vi "4155C PulsedStressV Config SMUs.vi"(0 "VISA resource name in":refnum<visa-resource-name>, 1 "Gate ON voltage":dbl min=-100.0 max=100.0 step=0.005 format="%.3f", 3 "Gate Standby":bool, 5 "Pulse period 2":dbl=0.05 min=0.005 max=1.0 step=0.0001 format="%.4f", 6 "SMU4":cluster{"on/off":bool, "Voltage":dbl} {"Voltage" min=-100.0 max=100.0 format="%.2f"}, 7 "Pulse width 2":dbl=0.0005 min=0.0005 max=0.1 step=0.0001 format="%.4f", 8 "Base voltage 2":dbl format="%^.4e", 11 "error in (no error)":errorcluster, 12 "Drain Voltage":dbl min=-100.0 max=100.0 step=0.005 format="%.3f", 14 "Drain Standby":bool) -> (4 "VISA Resource Name out":refnum<visa-resource-name>, 15 "error out":errorcluster)   [LabVIEW 2016]
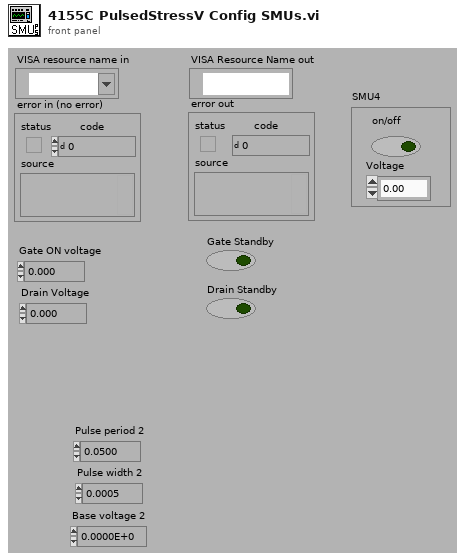
[diagram p1: front panel]
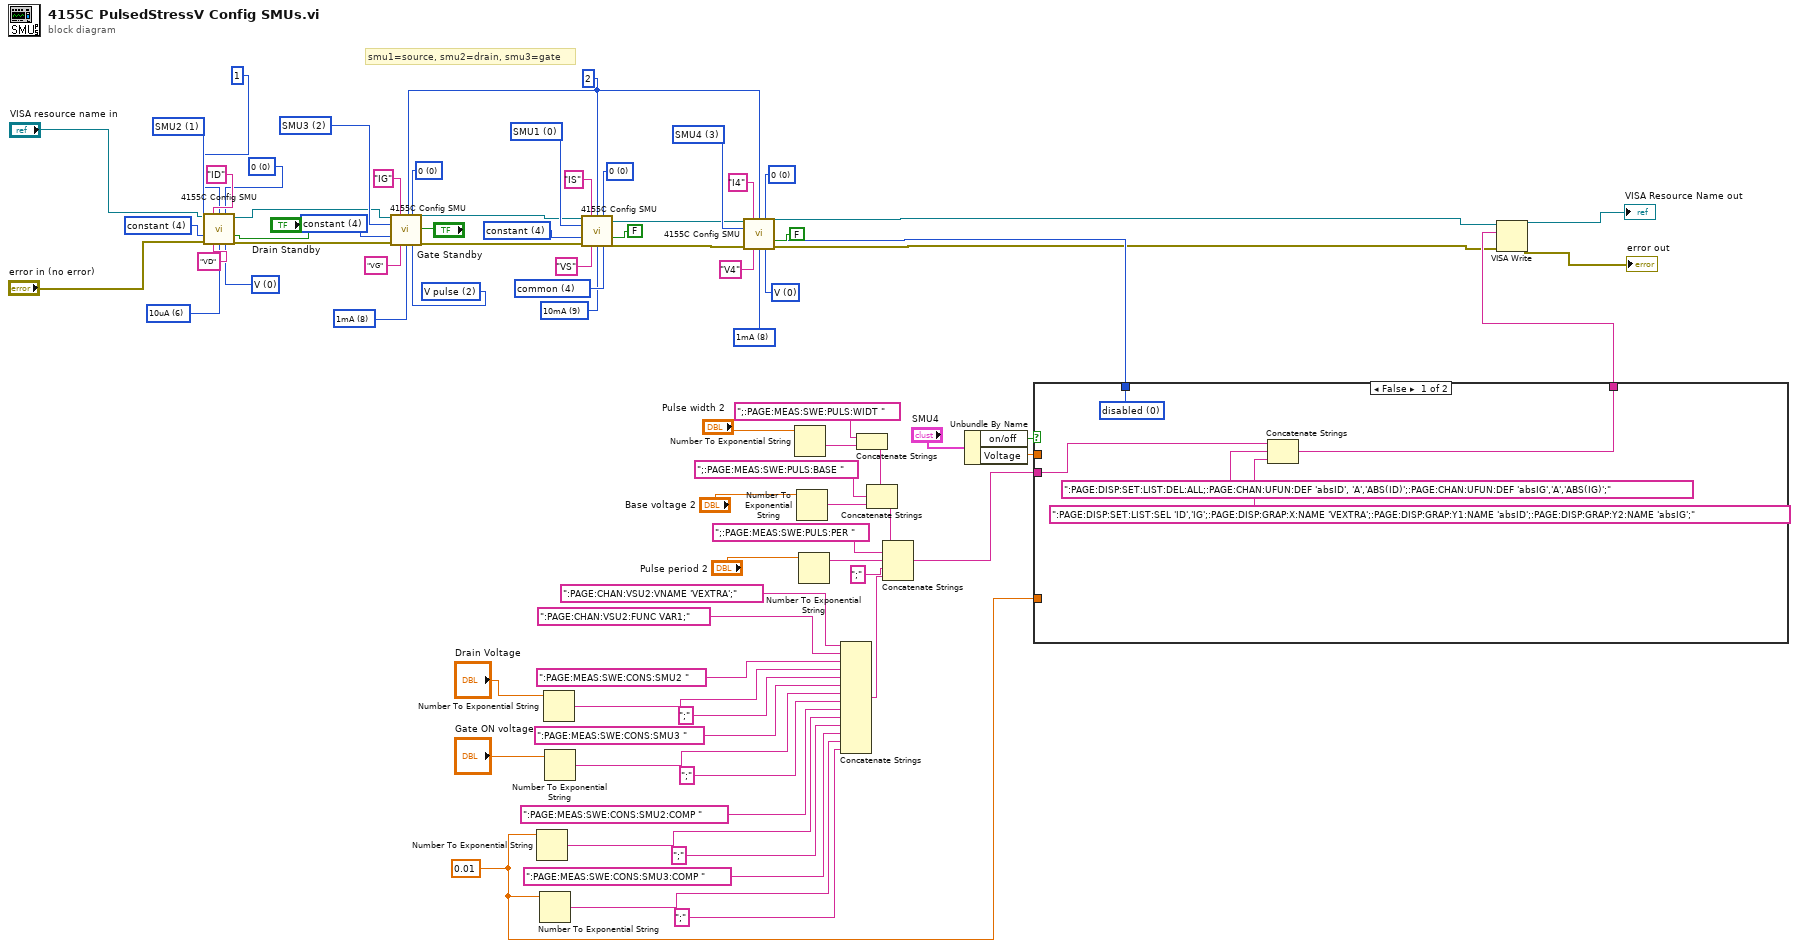
[diagram p0: block diagram]
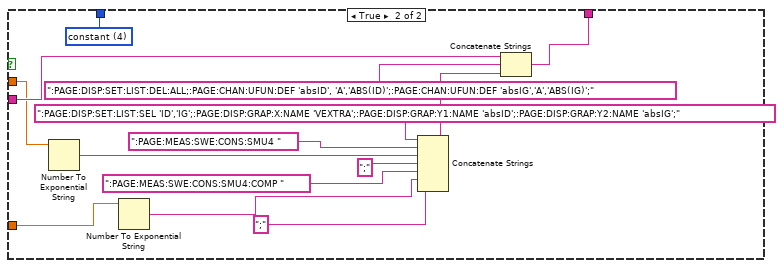
[diagram p2: hidden frame]
diagram:
  w13 = u8 6 items=["10pA  ", "100pA  ", "1nA  ", "10nA", "100nA", "1uA", "10uA", "100uA", "1mA", "10mA", "100mA", "1A"] ("Range")
  w18 = u8 8 items=["10pA  ", "100pA  ", "1nA  ", "10nA", "100nA", "1uA", "10uA", "100uA", "1mA", "10mA", "100mA", "1A"] ("Range")
  w22 = u8 8 items=["10pA  ", "100pA  ", "1nA  ", "10nA", "100nA", "1uA", "10uA", "100uA", "1mA", "10mA", "100mA", "1A"] ("Range")
  w23 = u32 2 items=["V  ", "I  ", "V pulse  ", "I pulse  ", "  common  "] ("mode")
  w21 = 2
  w24 = u8 9 items=["10pA  ", "100pA  ", "1nA  ", "10nA", "100nA", "1uA", "10uA", "100uA", "1mA", "10mA", "100mA", "1A"] ("Range")
  w9 = u32 1 items=["SMU1  ", "SMU2  ", "SMU3  ", "SMU4  ", "SMU5  ", "SMU6  "] ("unit to configure")
  w10 = u32 4 items=["disabled  ", "VAR1  ", "VAR2  ", "VAR1'  ", "constant  "] ("function")
  w6 = u32 0 items=["0  ", "10K Ohms  ", "100K Ohms  ", "1M Ohms  "] ("series resistance *")
  w12 = u32 0 items=["V  ", "I  ", "V pulse  ", "I pulse  ", "  common  "] ("mode")
  w29 = u32 0 items=["V  ", "I  ", "V pulse  ", "I pulse  ", "  common  "] ("mode")
  w30 = u32 0 items=["0  ", "10K Ohms  ", "100K Ohms  ", "1M Ohms  "] ("series resistance *")
  w32 = u32 3 items=["SMU1  ", "SMU2  ", "SMU3  ", "SMU4  ", "SMU5  ", "SMU6  "] ("unit to configure")
  w35 = u32 0 items=["0  ", "10K Ohms  ", "100K Ohms  ", "1M Ohms  "] ("series resistance *")
  w25 = u32 4 items=["disabled  ", "VAR1  ", "VAR2  ", "VAR1'  ", "constant  "] ("function")
  w37 = u32 2 items=["SMU1  ", "SMU2  ", "SMU3  ", "SMU4  ", "SMU5  ", "SMU6  "] ("unit to configure")
  w40 = u32 4 items=["V  ", "I  ", "V pulse  ", "I pulse  ", "  common  "] ("mode")
  w41 = u32 0 items=["0  ", "10K Ohms  ", "100K Ohms  ", "1M Ohms  "] ("series resistance *")
  w43 = u32 4 items=["disabled  ", "VAR1  ", "VAR2  ", "VAR1'  ", "constant  "] ("function")
  w44 = u32 0 items=["SMU1  ", "SMU2  ", "SMU3  ", "SMU4  ", "SMU5  ", "SMU6  "] ("unit to configure")
  w45 = 0.01 ("DRAIN CURRENT compliance")
  # "smu1=source, smu2=drain, smu3=gate"
  n1 = call "4155C Config SMU.vi"("VISA session"="VISA resource name in", "I name (max 6 chars)"="ID", "Range mode"=1, "series resistance *"=w6, "unit to configure"=w9, "function"=w10, "standby"="Drain Standby", "error in (no error)"="error in (no error)", "V name (max 6 chars)"="VD", "Range"=w13, "mode"=w12) -> ("dup VISA resource name"=w17:refnum<visa-resource-name>, "error out"=w15:errorcluster)  [unwired: 3 in]
  n2 = call "4155C Config SMU.vi"("VISA session"=w17, "I name (max 6 chars)"="IG", "Range mode"=w21, "series resistance *"=w35, "unit to configure"=w37, "function"=w25, "standby"="Gate Standby", "error in (no error)"=w15, "V name (max 6 chars)"="VG", "Range"=w22, "mode"=w23) -> ("dup VISA resource name"=w26:refnum<visa-resource-name>, "error out"=w16:errorcluster)  [unwired: 3 in]
  n3 = Number To Exponential String(number=w45) -> (E-format string=w50:string)  [unwired: 3 in]
  n4 = Number To Exponential String(number=w45) -> (E-format string=w47:string)  [unwired: 3 in]
  n5 = Number To Exponential String(number="Drain Voltage") -> (E-format string=w58:string)  [unwired: 3 in]
  n6 = Number To Exponential String(number="Gate ON voltage") -> (E-format string=w55:string)  [unwired: 3 in]
  n7 = call "4155C Config SMU.vi"("VISA session"=w26, "I name (max 6 chars)"="IS", "Range mode"=w21, "series resistance *"=w41, "unit to configure"=w44, "function"=w43, "standby"=FALSE, "error in (no error)"=w16, "V name (max 6 chars)"="VS", "Range"=w24, "mode"=w40) -> ("dup VISA resource name"=w20:refnum<visa-resource-name>, "error out"=w19:errorcluster)  [unwired: 3 in]
  n8 = Number To Exponential String(number="Pulse width 2") -> (E-format string=w72:string)  [unwired: 3 in]
  n9 = Number To Exponential String(number="Base voltage 2") -> (E-format string=w68:string)  [unwired: 3 in]
  n10 = Number To Exponential String(number="Pulse period 2") -> (E-format string=w65:string)  [unwired: 3 in]
  n11 = Concatenate Strings(":PAGE:CHAN:VSU2:VNAME 'VEXTRA';", ":PAGE:CHAN:VSU2:FUNC VAR1;", ":PAGE:MEAS:SWE:CONS:SMU2 " ("write buffer (\"\")"), w58, ";" ("Substring"), ":PAGE:MEAS:SWE:CONS:SMU3 " ("write buffer (\"\")"), w55, ";" ("Substring"), ":PAGE:MEAS:SWE:CONS:SMU2:COMP ", w50, ";" ("Substring"), ":PAGE:MEAS:SWE:CONS:SMU3:COMP ", w47, ";" ("Substring")) -> (w60:string)
  n12 = Concatenate Strings(";:PAGE:MEAS:SWE:PULS:WIDT " ("Substring"), w72) -> (w70:string)
  n13 = Concatenate Strings(w70, ";:PAGE:MEAS:SWE:PULS:BASE " ("Substring"), w68) -> (w66:string)
  n14 = Concatenate Strings(w66, ";:PAGE:MEAS:SWE:PULS:PER " ("Substring"), w65, ";" ("Substring"), w60) -> (w63:string)
  n15 = Unbundle By Name("SMU4") -> ("on/off"=w78:bool, "Voltage"=w79:dbl)
  n16 = case shown="False" w78 {
    tunnel: w63 -> [w86 w100]
    tunnel: [w85 w99] -> w76
    tunnel: w79 -> [_ w97]
    tunnel: [w84 w98] -> w2
    tunnel: w45 -> [_ w89]
    frame False {
      w84 = u32 0 items=["disabled  ", "VAR1  ", "VAR2  ", "VAR1'  ", "constant  "] ("function")
      n17 = Concatenate Strings(w86, ":PAGE:DISP:SET:LIST:DEL:ALL;:PAGE:CHAN:UFUN:DEF 'absID', 'A','ABS(ID)';:PAGE:CHAN:UFUN:DEF 'absIG','A','ABS(IG)';", ":PAGE:DISP:SET:LIST:SEL 'ID','IG';:PAGE:DISP:GRAP:X:NAME 'VEXTRA';:PAGE:DISP:GRAP:Y1:NAME 'absID';:PAGE:DISP:GRAP:Y2:NAME 'absIG';" ("write buffer (\"\")")) -> (w85:string)
    }
    frame True {
      w98 = u32 4 items=["disabled  ", "VAR1  ", "VAR2  ", "VAR1'  ", "constant  "] ("function")
      n18 = Number To Exponential String(number=w97) -> (E-format string=w95:string)  [unwired: 3 in]
      n19 = Number To Exponential String(number=w89) -> (E-format string=w91:string)  [unwired: 3 in]
      n20 = Concatenate Strings(":PAGE:DISP:SET:LIST:SEL 'ID','IG';:PAGE:DISP:GRAP:X:NAME 'VEXTRA';:PAGE:DISP:GRAP:Y1:NAME 'absID';:PAGE:DISP:GRAP:Y2:NAME 'absIG';" ("write buffer (\"\")"), ":PAGE:MEAS:SWE:CONS:SMU4 " ("write buffer (\"\")"), w95, ";" ("Substring"), ":PAGE:MEAS:SWE:CONS:SMU4:COMP ", w91, ";" ("Substring")) -> (w87:string)
      n21 = Concatenate Strings(w100, ":PAGE:DISP:SET:LIST:DEL:ALL;:PAGE:CHAN:UFUN:DEF 'absID', 'A','ABS(ID)';:PAGE:CHAN:UFUN:DEF 'absIG','A','ABS(IG)';", w87) -> (w99:string)
    }
  }
  n22 = call "4155C Config SMU.vi"("VISA session"=w20, "I name (max 6 chars)"="I4", "Range mode"=w21, "series resistance *"=w30, "unit to configure"=w32, "function"=w2, "standby"=FALSE, "error in (no error)"=w19, "V name (max 6 chars)"="V4", "Range"=w18, "mode"=w29) -> ("dup VISA resource name"=w3:refnum<visa-resource-name>, "error out"=w1:errorcluster)  [unwired: 3 in]
  n23 = VISA Write(VISA resource name=w3, write buffer=w76, error in (no error)=w1) -> (VISA resource name out=→"VISA Resource Name out":refnum<visa-resource-name>, error out=→"error out":errorcluster)  [unwired: 1 out]
